vi "IntuitiveSteering_main.vi"(8 "Error In":errorcluster, 10 "dt":dbl, 11 "Time In":dbl format="%#_13g") -> (0 "Error Out":errorcluster, 2 "Servo Position":T1, 3 "Time Out":dbl)   [LabVIEW 2013]
uses:
  My Computer/Controls/Servo Position.ctl
  My Computer/Controls/Intuitive Steering.ctl
  My Computer/Controls/Steering Inputs.ctl
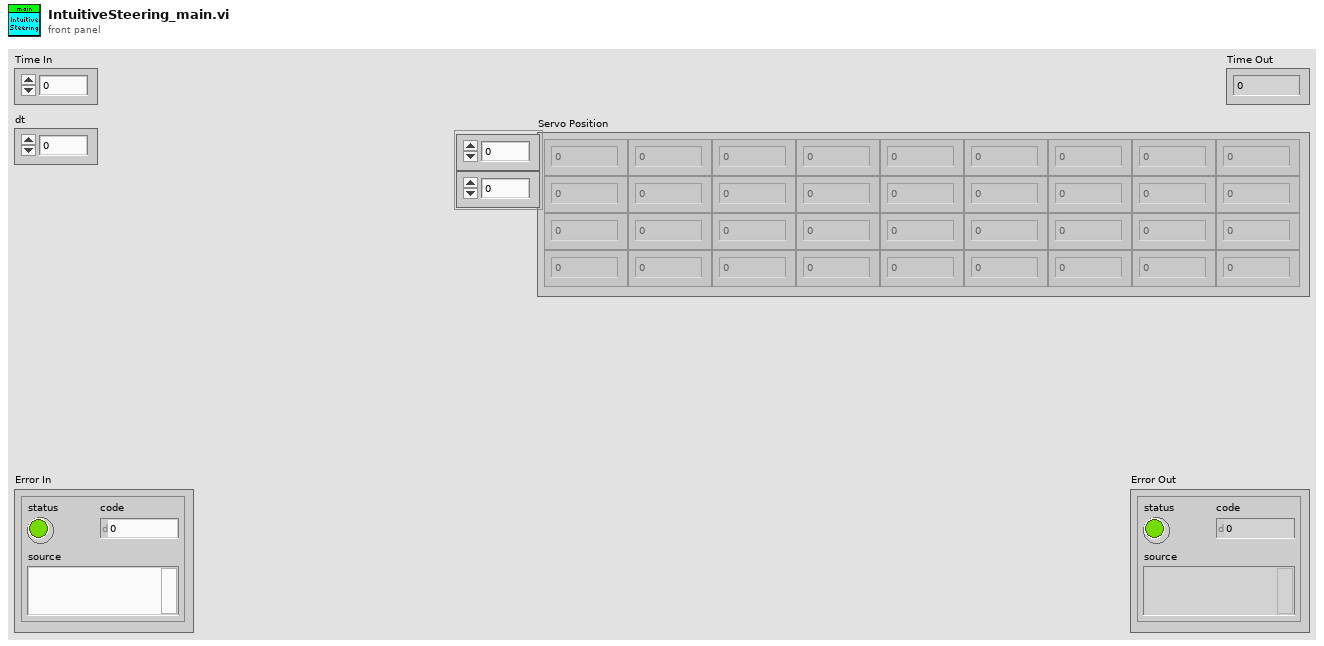
[diagram p1: front panel]
types:
  T1 = typedef "Servo Position.ctl" = dbl[][]
  T2 = typedef "Intuitive Steering.ctl" = cluster{"Frequency (Hz):":dbl, "Max. Amplitude (°):":dbl, "Phase Shift (/Pi):":dbl, "Flap (°):":dbl, "Flap Saturation:":dbl}
  T3 = typedef "Steering Inputs.ctl" = cluster{"X":dbl, "Y":dbl, "Z":dbl, "phi":dbl, "theta":dbl, "psi":dbl}
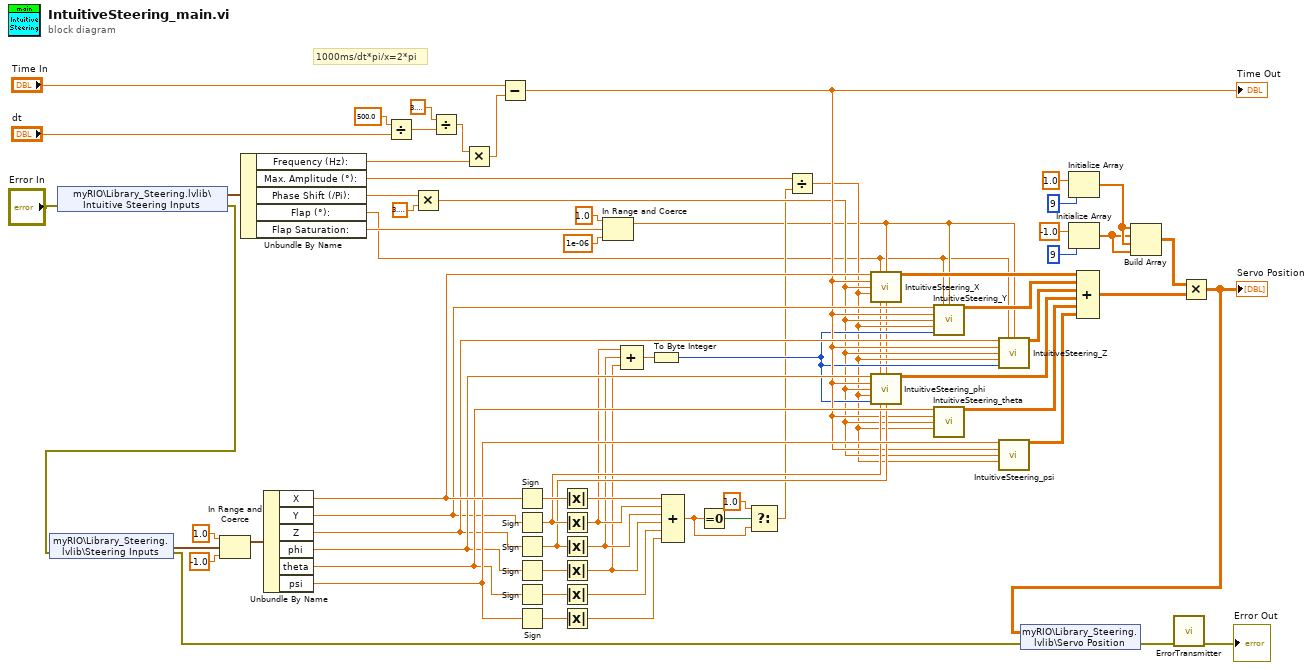
[diagram p0: block diagram]
diagram:
  # "1000ms/dt*pi/x=2*pi"
  n1 = shared-variable "myRIO\\Library_Steering.lvlib\\Intuitive Steering Inputs"(error in="Error In") -> (w11:T2, error out=w28:errorcluster)
  n2 = shared-variable "myRIO\\Library_Steering.lvlib\\Steering Inputs"(error in=w28) -> (w2:T3, error out=w27:errorcluster)
  n3 = In Range and Coerce(upper limit=1.0, x=w2, lower limit=-1.0) -> (coerced(x)=w1:T3)  [unwired: 1 out]
  n4 = Unbundle By Name(w11) -> ("Frequency (Hz):"=w10:dbl, "Max. Amplitude (°):"=w9:dbl, "Phase Shift (/Pi):"=w8:dbl, "Flap (°):"=w5:dbl, "Flap Saturation:"=w7:dbl)
  n5 = Unbundle By Name(w1) -> ("X"=w53:dbl, "Y"=w37:dbl, "Z"=w45:dbl, "phi"=w46:dbl, "theta"=w47:dbl, "psi"=w48:dbl)
  n6 = Divide(x=500.0, y="dt") -> (x/y=w12:dbl)
  n7 = Multiply(x=w8, y=3.141592653589793) -> (x*y=w34:dbl)
  n8 = Divide(x=3.141592653589793, y=w12) -> (x/y=w63:dbl)
  n9 = Multiply(x=w63, y=w10) -> (x*y=w62:dbl)
  n10 = Subtract(x="Time In", y=w62) -> (x-y=w36:dbl)
  "Time Out" <- w36
  n11 = Sign(1:w53) -> (0:w61:dbl)
  n12 = Sign(1:w37) -> (0:w44:dbl)
  n13 = Sign(1:w45) -> (0:w43:dbl)
  n14 = Sign(1:w46) -> (0:w59:dbl)
  n15 = Sign(1:w47) -> (0:w58:dbl)
  n16 = Sign(1:w48) -> (0:w57:dbl)
  n17 = Absolute Value(x=w61) -> (abs(x)=w60:dbl)
  n18 = Absolute Value(x=w44) -> (abs(x)=w41:dbl)
  n19 = Absolute Value(x=w43) -> (abs(x)=w40:dbl)
  n20 = Absolute Value(x=w59) -> (abs(x)=w39:dbl)
  n21 = Absolute Value(x=w58) -> (abs(x)=w55:dbl)
  n22 = Absolute Value(x=w57) -> (abs(x)=w56:dbl)
  n23 = In Range and Coerce(upper limit=1.0, x=w7, lower limit=1e-06) -> (coerced(x)=w6:dbl)  [unwired: 1 out]
  n24 = Compound Arithmetic op=ADD(w41, w40, w39) -> (w42:dbl)
  n25 = To Byte Integer(number=w42) -> (8bit integer=w35:i8)
  n26 = Compound Arithmetic op=ADD(w60, w41, w40, w39, w55, w56) -> (w31:dbl)
  n27 = Equal To 0?(x=w31) -> (x = 0?=w33:bool)
  n28 = Select(t=1.0, s=w33, f=w31) -> (s? t:f=w29:dbl)
  n29 = Divide(x=w9, y=w29) -> (x/y=w30:dbl)
  n30 = call "IntuitiveSteering_X.vi"("Input"=w53, "Forward Time"=w36, "Phase Shift"=w34, "Max. Amplitude"=w30) -> ("Servo Position"=w54:T1)  [unwired: 11 in]
  n31 = call "IntuitiveSteering_phi.vi"("Input"=w46, "Flap"=w5, "Flap Saturation"=w6, "Forward Time"=w36, "Phase Shift"=w34, "Max. Amplitude"=w30, "nonZeroPositionIndex"=w35, "WhatDoesY"=w44, "WhatDoesZ"=w43) -> ("Servo Position"=w51:T1)  [unwired: 6 in]
  n32 = call "IntuitiveSteering_Y.vi"("Input"=w37, "Flap"=w5, "Flap Saturation"=w6, "Forward Time"=w36, "Phase Shift"=w34, "Max. Amplitude"=w30, "nonZeroPositionIndex"=w35) -> ("Servo Position"=w38:T1)  [unwired: 8 in]
  n33 = call "IntuitiveSteering_theta.vi"("Input"=w47, "Forward Time"=w36, "Phase Shift"=w34, "Max. Amplitude"=w30) -> ("Servo Position"=w50:T1)  [unwired: 11 in]
  n34 = call "IntuitiveSteering_Z.vi"("Input"=w45, "Flap"=w5, "Flap Saturation"=w6, "Forward Time"=w36, "Phase Shift"=w34, "Max. Amplitude"=w30, "nonZeroPositionIndex"=w35) -> ("Servo Position"=w52:T1)  [unwired: 8 in]
  n35 = call "IntuitiveSteering_psi.vi"("Input"=w48, "Forward Time"=w36, "Phase Shift"=w34, "Max. Amplitude"=w30) -> ("Servo Position"=w49:T1)  [unwired: 11 in]
  n36 = Initialize Array(1.0 ("element"), 9 ("dimension size")) -> (w20:dbl[])
  n37 = Initialize Array(-1.0 ("element"), 9 ("dimension size")) -> (w19:dbl[])
  n38 = Compound Arithmetic op=ADD(w54, w38, w52, w51, w50, w49) -> (w18:T1)
  n39 = Build Array(w20, w19, w20, w19) -> (w16:dbl[][])
  n40 = Multiply(x=w16, y=w18) -> (x*y=w17:T1)
  "Servo Position" <- w17
  n41 = shared-variable "myRIO\\Library_Steering.lvlib\\Servo Position"(w17, error in=w27) -> (error out=w15:errorcluster)
  n42 = call "ErrorTransmitter.vi"("Error In"=w15) -> ("Error Out"=→"Error Out":errorcluster)  [unwired: 10 in]
